vi "GDX_UsbAndBluetooth.vi"() -> ()   [LabVIEW 2019]
panel:
  out "subarray":dbl[](array[numeric])
  out "Waveform Chart":dbl[][](graph)
  out "XY Graph 2":cluster{dbl[], dbl[]}[](graph)
  out "XY Graph":cluster{dbl[], dbl[]}[](graph)
  in  "stop":bool
  out "error out":errorcluster
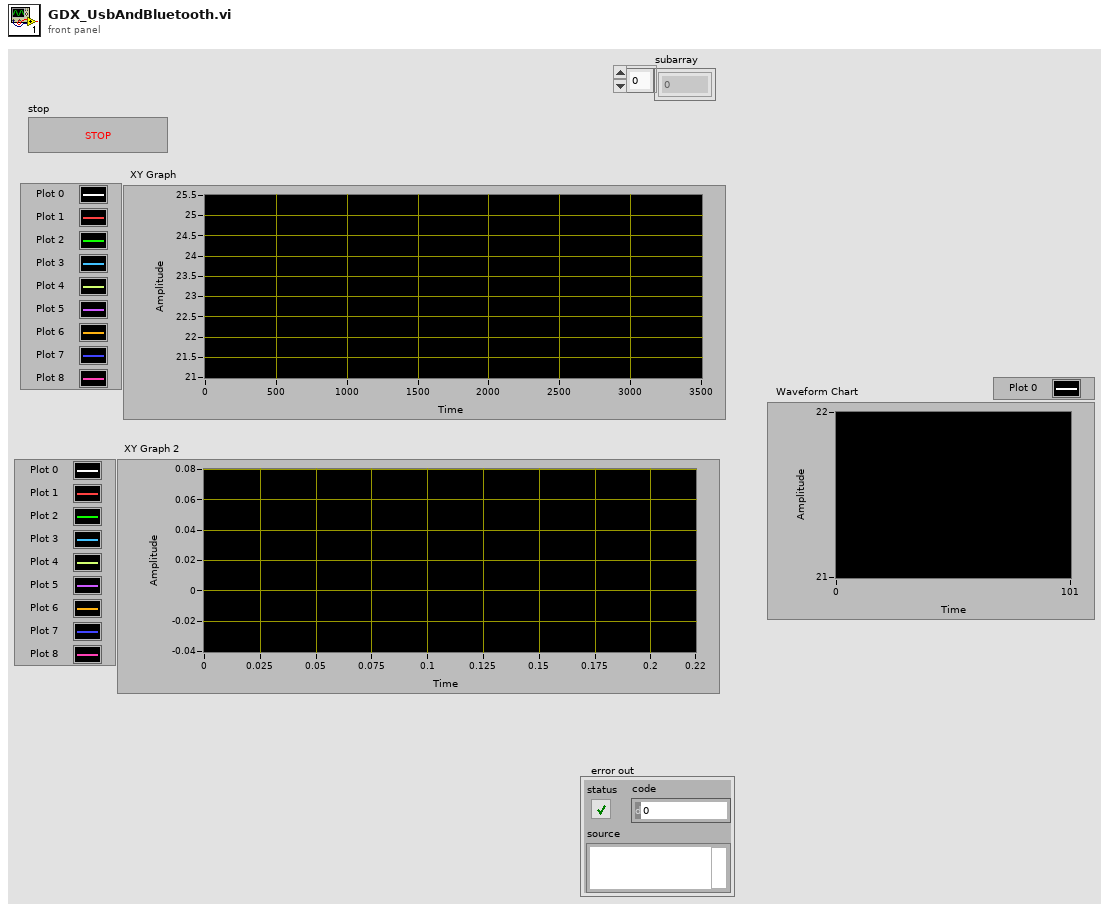
[diagram p1: front panel]
types:
  T1 = typedef "D2PIO_D2PIOCluster.ctl" = cluster{"Library Handle":i64, "Device List Handle":i64, "BT Device Handles":i64[], "USB Device Handles":i64[], "BT+USB Device Handles":i64[], "Measurement Tick":dbl[], "Ch Availability Mask":u32[]}
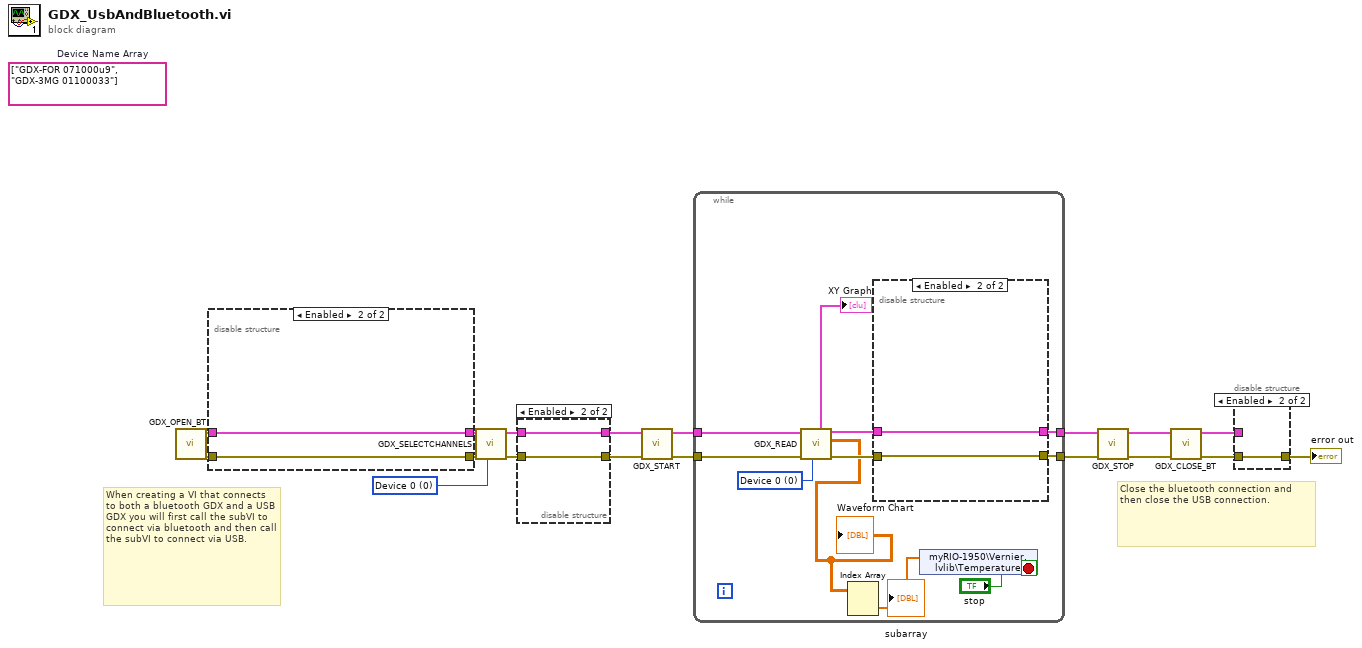
[diagram p0: block diagram]
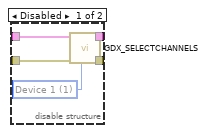
[diagram p2: hidden frame]
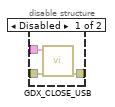
[diagram p3: hidden frame]
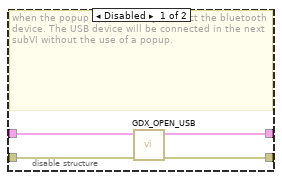
[diagram p4: hidden frame]
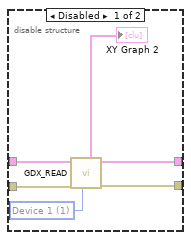
[diagram p5: hidden frame]
diagram:
  w1 = 0 items=["Device 0", "Device 1", "Device 2", "Device 3", "Device 4", "Device 5", "Device 6", "Device 7", "Device 8", "Device 9", "Device 10", "Device 11"] ("Device Index")
  (unwired) string[] ["GDX-FOR 071000u9", "GDX-3MG 01100033"]  # Device Name Array
  # "Close the bluetooth connection and then close the USB connection."
  # "When creating a VI that connects to both a bluetooth GDX and a USB GDX you will first call the subVI to connect via bluetooth and then call the subVI to connect via USB."
  n1 = call <vilib>:"GDX_OPEN_BT.vi"() -> ("error out"=w13:errorcluster, "D2PIO Cluster Out"=w14:T1)  [unwired: 10 in]
  n2 = disable-structure shown="Enabled" {
    disable-tunnel: w14 -> [w22 w23]
    disable-tunnel: w13 -> [w21 w24]
    disable-tunnel: [w20 w23] -> w12
    disable-tunnel: [w19 w24] -> w11
    frame Disabled {
      # "when the popup appears, only connect the bluetooth device. The USB device will be connected in the next subVI without the use of a popup."
      n3 = call <vilib>:"GDX_OPEN_USB.vi"("error in (no error)"=w21, "D2PIO Cluster In"=w22) -> ("error out"=w19:errorcluster, "D2PIO Cluster Out"=w20:T1)  [unwired: 7 in, 1 out]
    }
    frame Enabled {
    }
  }
  n4 = call <vilib>:"GDX_SELECTCHANNELS.vi"("Device Index"=w1, "error in (no error)"=w11, "D2PIO Cluster In"=w12) -> ("error out"=w4:errorcluster, "D2PIO Cluster Out"=w5:T1)  [unwired: 7 in]
  n5 = disable-structure shown="Enabled" {
    disable-tunnel: w5 -> [w29 w30]
    disable-tunnel: w4 -> [w28 w31]
    disable-tunnel: [w27 w31] -> w3
    disable-tunnel: [w26 w30] -> w2
    frame Disabled {
      w25 = 1 items=["Device 0", "Device 1", "Device 2", "Device 3", "Device 4", "Device 5", "Device 6", "Device 7", "Device 8", "Device 9", "Device 10", "Device 11"] ("Device Index")
      n6 = call <vilib>:"GDX_SELECTCHANNELS.vi"("Device Index"=w25, "error in (no error)"=w28, "D2PIO Cluster In"=w29) -> ("error out"=w27:errorcluster, "D2PIO Cluster Out"=w26:T1)  [unwired: 7 in]
    }
    frame Enabled {
    }
  }
  n7 = call <vilib>:"GDX_START.vi"("error in (no error)"=w3, "D2PIO Cluster In"=w2) -> ("error out"=w18:errorcluster, "D2PIO Cluster Out"=w17:T1)  [unwired: 6 in, 2 out]
  n8 = while {
    tunnel: w18 -> [w42]
    tunnel: w17 -> [w40]
    tunnel: [w37] -> w16
    tunnel: [w36] -> w15
    stop <- "stop" stop-if-true
    w35 = 0 items=["Device 0", "Device 1", "Device 2", "Device 3", "Device 4", "Device 5", "Device 6", "Device 7", "Device 8", "Device 9", "Device 10", "Device 11"] ("Device Index")
    n9 = call <vilib>:"GDX_READ.vi"("Device Index"=w35, "error in (no error)"=w42, "D2PIO Cluster In"=w40) -> ("error out"=w39:errorcluster, "Waveform Chart Data"=w33:dbl[][], "D2PIO Cluster Out"=w38:T1, "XY Graph Data"=→"XY Graph":cluster{dbl[], dbl[]}[])  [unwired: 3 in, 2 out]
    "Waveform Chart" <- w33
    n10 = Index Array(array=w33) -> (element=w32:dbl[])  [unwired: 2 in]
    "subarray" <- w32
    n11 = disable-structure shown="Enabled" {
      disable-tunnel: w39 -> [w48 w49]
      disable-tunnel: w38 -> [w47 w50]
      disable-tunnel: [w46 w50] -> w37
      disable-tunnel: [w45 w49] -> w36
      frame Disabled {
        w43 = 1 items=["Device 0", "Device 1", "Device 2", "Device 3", "Device 4", "Device 5", "Device 6", "Device 7", "Device 8", "Device 9", "Device 10", "Device 11"] ("Device Index")
        n12 = call <vilib>:"GDX_READ.vi"("Device Index"=w43, "error in (no error)"=w48, "D2PIO Cluster In"=w47) -> ("error out"=w45:errorcluster, "D2PIO Cluster Out"=w46:T1, "XY Graph Data"=→"XY Graph 2":cluster{dbl[], dbl[]}[])  [unwired: 3 in, 3 out]
      }
      frame Enabled {
      }
    }
    n13 = shared-variable "myRIO-1950\\Vernier.lvlib\\Temperature"(w32) -> ()  [unwired: 1 in, 1 out]
  }
  n14 = call <vilib>:"GDX_STOP.vi"("error in (no error)"=w15, "D2PIO Cluster In"=w16) -> ("error out"=w10:errorcluster, "D2PIO Cluster Out"=w9:T1)  [unwired: 8 in]
  n15 = call <vilib>:"GDX_CLOSE_BT.vi"("error in (no error)"=w10, "D2PIO Cluster In"=w9) -> ("error out"=w7:errorcluster, "D2PIO Cluster Out"=w8:T1)  [unwired: 8 in]
  n16 = disable-structure shown="Enabled" {
    disable-tunnel: w8 -> [w53 _]
    disable-tunnel: w7 -> [w52 w54]
    disable-tunnel: [w51 w54] -> w6
    frame Disabled {
      n17 = call <vilib>:"GDX_CLOSE_USB.vi"("error in (no error)"=w52, "D2PIO Cluster In"=w53) -> ("error out"=w51:errorcluster)  [unwired: 8 in, 1 out]
    }
    frame Enabled {
    }
  }
  "error out" <- w6
